vi "PWM Pulsate (Direct).vi"() -> ()   [LabVIEW 2020, in "CTI-Scratchpad.lvlib"]
uses:
  CTI-Scratchpad.lvlib
  CTI/GPIO Number.ctl
  CTI/VisaComms/VisaComms.lvclass
  <vilib>/ptbypt/NI_PtbyPt.lvlib
  CTI/CTI.lvlib
panel:
  in  "Speed":i32(slide) scale=1000.0..1.0
  in  "stop":bool
  out "Act. Duty":sgl format="%_6f"
  in  "Port":refnum<visa-resource-name>="COM3"
  in  "Channel":T1
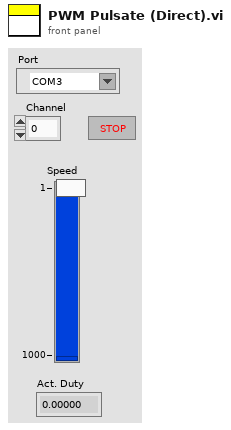
[diagram p1: front panel]
types:
  T1 = typedef "CTI.lvlib/GPIO Number.ctl" = i8
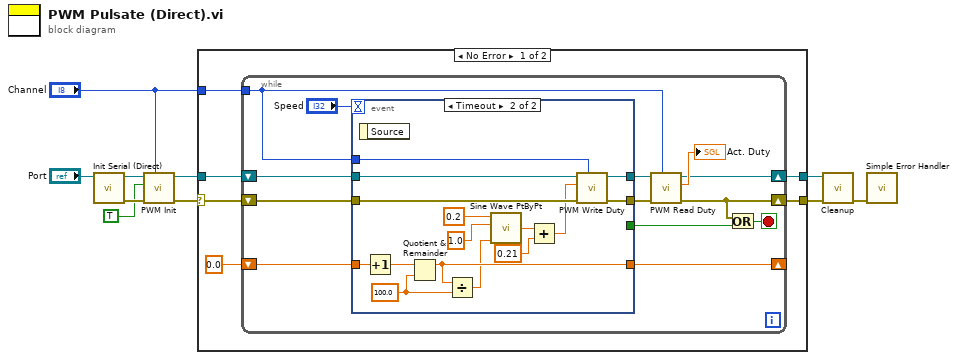
[diagram p0: block diagram]
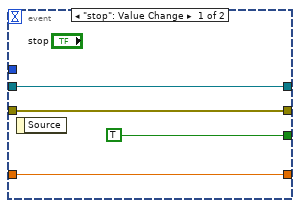
[diagram p2: hidden frame]
diagram:
  n1 = call "Init Serial (Direct).vi"("VISA resource name in"="Port") -> ("error out"=w8:errorcluster, "VisaComms out"=w9:refnum<class "VisaComms.lvclass">)  [unwired: 8 in, 1 out]
  n2 = call-dynamic "PWM Init.vi"("GPIO #"="Channel", "error in (no error)"=w8, "Enable (F)"=TRUE, "VisaComms in"=w9) -> ("error out"=w7:errorcluster, "VisaComms out"=w6:refnum<class "VisaComms.lvclass">)  [unwired: 6 in]
  n3 = case shown="No Error" w7 {
    selector: w7 -> [w15 w49]
    tunnel: w6 -> [w16 w50]
    tunnel: [w14 w50] -> w4
    tunnel: [w13 w49] -> w5
    tunnel: "Channel" -> [w12 _]
    frame No Error {
      n4 = while {
        shift-right: [w21] -> w14
        shift-left: w16 -> [w28]
        shift-right: [w20] -> w13
        shift-left: w15 -> [w27]
        tunnel: w12 -> [w17]
        shift-right: [w18] -> _
        shift-left: 0.0 -> [w19]
        stop <- w29 stop-if-true
        n5 = event shown="[1] Timeout" {
          selector: _ -> [_ _]
          dyn-events: _ -> [_ _]
          timeout: "Speed" -> [_ _]
          tunnel: [w33 w41] -> w25
          tunnel: w28 -> [w33 w46]
          tunnel: [w32 w42] -> w24
          tunnel: w27 -> [w32 w45]
          tunnel: [TRUE _] -> w26
          tunnel: w19 -> [w30 w40]
          tunnel: [w30 w37] -> w18
          tunnel: w17 -> [_ w35]
          event "stop": Value Change {
            n6 = event-data() -> ()  [unwired: 1 in, 1 out]
          }
          event Timeout {
            w38 = 100.0 ("frequency")
            n7 = event-data() -> ()  [unwired: 1 in, 1 out]
            n8 = Increment(x=w40) -> (x+1=w39:dbl)
            n9 = Quotient & Remainder(x=w39, y=w38) -> (x-y*floor(x/y)=w37:dbl)  [unwired: 1 out]
            n10 = Divide(x=w37, y=w38) -> (x/y=w36:dbl)
            n11 = call <vilib>:"Sine Wave PtByPt.vi"("time"=w36, "frequency"=1.0, "amplitude"=0.2) -> ("sine wave"=w44:dbl)  [unwired: 1 in]
            n12 = Add(x=w44, y=0.21) -> (x+y=w34:dbl)
            n13 = call-dynamic "PWM Write Duty.vi"("GPIO #"=w35, "error in (no error)"=w45, "Duty % (0-1)"=w34, "VisaComms in"=w46) -> ("error out"=w42:errorcluster, "VisaComms out"=w41:refnum<class "VisaComms.lvclass">)  [unwired: 6 in]
          }
        }
        n14 = call-dynamic "PWM Read Duty.vi"("GPIO #"=w17, "error in (no error)"=w24, "VisaComms in"=w25) -> ("error out"=w20:errorcluster, "Duty % (0-1)"=→"Act. Duty":sgl, "VisaComms out"=w21:refnum<class "VisaComms.lvclass">)  [unwired: 6 in]
        n15 = Or(x=w20, y=w26) -> (x .or. y?=w29:bool)
      }
    }
    frame Error {
    }
  }
  n16 = call-dynamic "Cleanup.vi"("error in (no error)"=w5, "VisaComms in"=w4) -> ("error out"=w3:errorcluster)  [unwired: 9 in]
  n17 = call <vilib>:"Simple Error Handler.vi"("error in (no error)"=w3) -> ()  [unwired: 4 in, 5 out]
